vi "parseReportServerIDResponse.vi"(8 "error in (no error)":errorcluster, 10 "DynamicFrameParser":refnum<class "DynamicFrameParser.lvclass">, 11 "ILC in":refnum<class "ILC.lvclass">) -> (0 "error out":errorcluster, 3 "ILC out":refnum<class "ILC.lvclass">)   [LabVIEW 2015, in "RTILC.lvlib" / "ILC.lvclass"]
uses:
  ILC.lvclass
  Common_RT_Modbus/DynamicFrameParser/DynamicFrameParser.lvclass
  Common_RT_Modbus/DataTypes/ExceptionCodes.ctl
  ILC.lvclass/ILC.ctl
  Common_RT_Modbus/RTModbus.lvlib
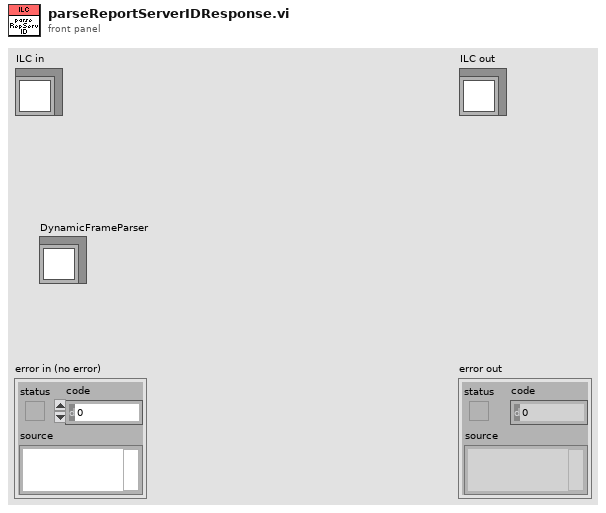
[diagram p1: front panel]
types:
  T1 = typedef "RTModbus.lvlib/ExceptionCodes.ctl" = u16
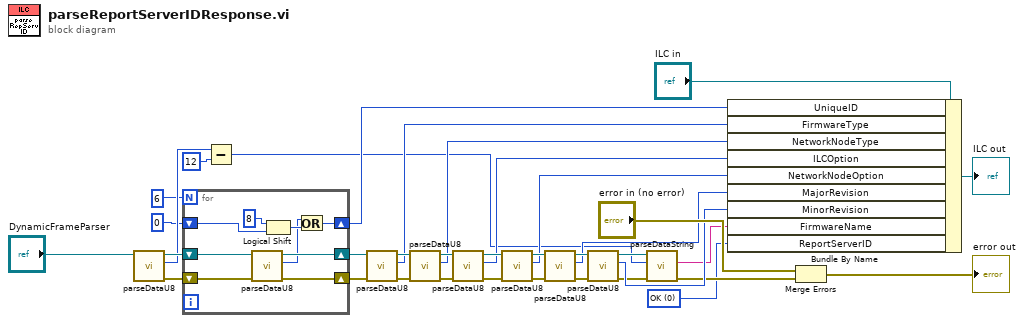
[diagram p0: block diagram]
diagram:
  w1 = T1 0 items=["OK", "IllegalFunction", "IllegalDataAddress", "IllegalDataValue", "SlaveDeviceFailure", "Acknowledge", "SlaveDeviceBusy", "NegativeAcknowledge", "MemoryParityError", "GatewayPathUnavailable", "GatewayTargetDeviceFailedToRespond"] ("ILCData.Responses.ReportServerID")
  n1 = call "parseDataU8.vi"("FrameParser in"="DynamicFrameParser") -> ("error out"=w30:errorcluster, "Data"=w29:u8, "FrameParser out"=w32:refnum<class "DynamicFrameParser.lvclass">)  [unwired: 8 in]
  n2 = for {
    N: 6 -> [_]
    shift-right: [w42] -> w15
    shift-left: w32 -> [w45]
    shift-right: [w37] -> w26
    shift-left: u64 0 -> [w41]
    shift-right: [w43] -> w14
    shift-left: w30 -> [w44]
    n3 = call "parseDataU8.vi"("error in (no error)"=w44, "FrameParser in"=w45) -> ("error out"=w43:errorcluster, "Data"=w38:u8, "FrameParser out"=w42:refnum<class "DynamicFrameParser.lvclass">)  [unwired: 7 in]
    n4 = Logical Shift(y=i16 8, x=w41) -> (x << y=w39:u64)
    n5 = Or(x=w38, y=w39) -> (x .or. y?=w37:u64)
  }
  n6 = Subtract(x=w29, y=u8 12) -> (x-y=w5:u8)
  n7 = call "parseDataU8.vi"("error in (no error)"=w14, "FrameParser in"=w15) -> ("error out"=w25:errorcluster, "Data"=w13:u8, "FrameParser out"=w24:refnum<class "DynamicFrameParser.lvclass">)  [unwired: 7 in]
  n8 = call "parseDataU8.vi"("error in (no error)"=w25, "FrameParser in"=w24) -> ("error out"=w23:errorcluster, "Data"=w12:u8, "FrameParser out"=w22:refnum<class "DynamicFrameParser.lvclass">)  [unwired: 7 in]
  n9 = call "parseDataU8.vi"("error in (no error)"=w23, "FrameParser in"=w22) -> ("error out"=w21:errorcluster, "Data"=w11:u8, "FrameParser out"=w20:refnum<class "DynamicFrameParser.lvclass">)  [unwired: 7 in]
  n10 = call "parseDataU8.vi"("error in (no error)"=w21, "FrameParser in"=w20) -> ("error out"=w19:errorcluster, "Data"=w10:u8, "FrameParser out"=w18:refnum<class "DynamicFrameParser.lvclass">)  [unwired: 7 in]
  n11 = call "parseDataU8.vi"("error in (no error)"=w19, "FrameParser in"=w18) -> ("error out"=w17:errorcluster, "Data"=w9:u8, "FrameParser out"=w16:refnum<class "DynamicFrameParser.lvclass">)  [unwired: 7 in]
  n12 = call "parseDataU8.vi"("error in (no error)"=w17, "FrameParser in"=w16) -> ("error out"=w6:errorcluster, "Data"=w8:u8, "FrameParser out"=w7:refnum<class "DynamicFrameParser.lvclass">)  [unwired: 7 in]
  n13 = call "parseDataString.vi"("error in (no error)"=w6, "Length"=w5, "FrameParser in"=w7) -> ("error out"=w3:errorcluster, "Data"=w4:string)  [unwired: 6 in, 1 out]
  n14 = Bundle By Name(cluster="ILC in", "UniqueID"=w26, "FirmwareType"=w13, "NetworkNodeType"=w12, "ILCOption"=w11, "NetworkNodeOption"=w10, "MajorRevision"=w9, "MinorRevision"=w8, "FirmwareName"=w4, "ReportServerID"=w1) -> (→"ILC out":refnum<class "ILC.lvclass">)
  n15 = Merge Errors("error in (no error)", w3) -> (→"error out":errorcluster)
